vi "StutterShifterState.vi"(9 "Requested Shifter State":bool, 10 "Request Stutter":bool) -> (0 "Stuttered Shifter State":bool)   [LabVIEW 2020]
doc: "This VI rapidly \"stutters\" the shifter in the event the sensors failed to detect a successful shift, in order to try and get the balls to engage."
panel:
  in  "Stutter Time":u32=100
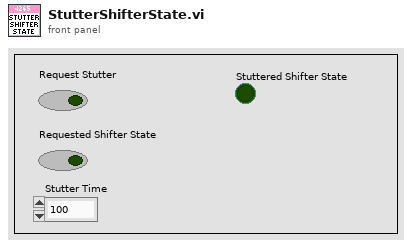
[diagram p1: front panel]
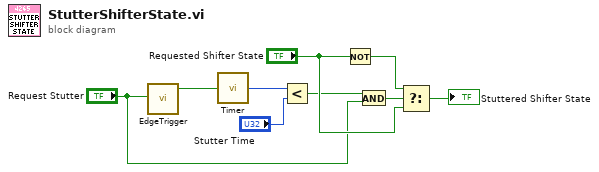
[diagram p0: block diagram]
diagram:
  n1 = call "EdgeTrigger.vi"("Input Signal"="Request Stutter") -> ("Rising Edge Trigger"=w9:bool)  [unwired: 2 out]
  n2 = call "Timer.vi"("Reset Timer"=w9) -> ("Time (ms)"=w8:u32)
  n3 = Less?(x=w8, y="Stutter Time") -> (x < y?=w4:bool)
  n4 = Not(x="Requested Shifter State") -> (.not. x?=w7:bool)
  n5 = And(x=w4, y="Request Stutter") -> (x .and. y?=w5:bool)
  n6 = Select(t=w7, s=w5, f="Requested Shifter State") -> (s? t:f=→"Stuttered Shifter State":bool)
